vi "Set LED colors.vi"(8 "error in":errorcluster, 9 "On color":i32=-1, 10 "Off color":i32=-1, 11 "reference":refnum<vi>) -> (0 "error out":errorcluster, 3 "reference out":refnum<vi>)   [LabVIEW 2020]
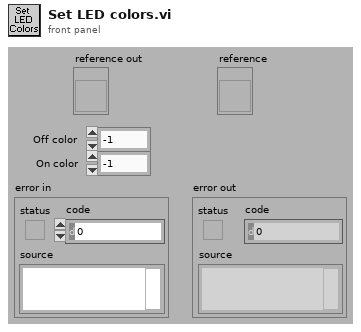
[diagram p1: front panel]
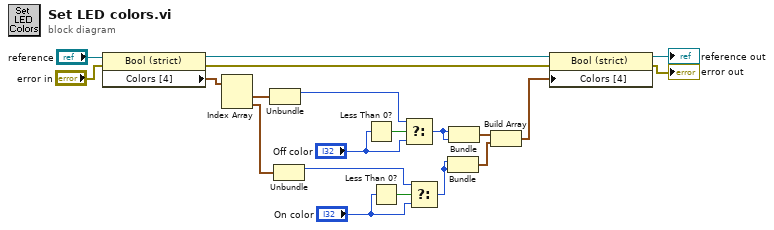
[diagram p0: block diagram]
diagram:
  n1 = property on="Property Node" class="Bool (strict)"(reference="reference", error in="error in") -> (reference out=w13:refnum<vi>, error out=w12:errorcluster, "Colors [4]"=w11:cluster{u32, u32}[])
  n2 = Index Array(array=w11) -> (element #1=w10:cluster{u32, u32}, element #2=w9:cluster{u32, u32})  [unwired: 2 in]
  n3 = Unbundle(w10) -> (w6:u32)  [unwired: 1 out]
  n4 = Unbundle(w9) -> (w2:u32)  [unwired: 1 out]
  n5 = Less Than 0?(x="Off color") -> (x < 0?=w8:bool)
  n6 = Less Than 0?(x="On color") -> (x < 0?=w4:bool)
  n7 = Select(t=w6, s=w8, f="Off color") -> (s? t:f=w5:u32)
  n8 = Select(t=w2, s=w4, f="On color") -> (s? t:f=w1:u32)
  n9 = Bundle("On color"=w1, "On color"=w1) -> (w18:cluster{"On color":u32, "On color":u32})  [unwired: 1 in]
  n10 = Bundle("Off color"=w5, "Off color"=w5) -> (w20:cluster{"Off color":u32, "Off color":u32})  [unwired: 1 in]
  n11 = Build Array(w20, w18) -> (w19:cluster{"On color":u32, "On color":u32}[])
  n12 = property on="Property Node" class="Bool (strict)"(reference=w13, error in=w12, "Colors [4]"=w19) -> (reference out=→"reference out":refnum<vi>, error out=→"error out":errorcluster)
